vi "CRYUpdate Jump Info Lib.vi"(0 "Steps In":T2[](array[typedef]) {"Repeat State Array"."Start" format="%#_5g"; "Y dB ref" format="%.1f"; "Y data" items=["dB", "Lin"]; "Start" format="%#_5g"}, 1 "sOption":string, 5 "Action":T3(ring), 7 "Step number Selected":i32, 9 "MoveCount":i32, 11 "SourceCount":i32) -> (4 "Steps Out":T2[](array[typedef]) {"Repeat State Array"."Start" format="%#_5g"; "Y dB ref" format="%.1f"; "Y data" items=["dB", "Lin"]; "Start" format="%#_5g"}, 6 "Jump State Out":T1(array[cluster]), 15 "Canceled?":bool)   [LabVIEW 2013]
uses:
  CRYSystem/Typedef Control/CRYStep.ctl
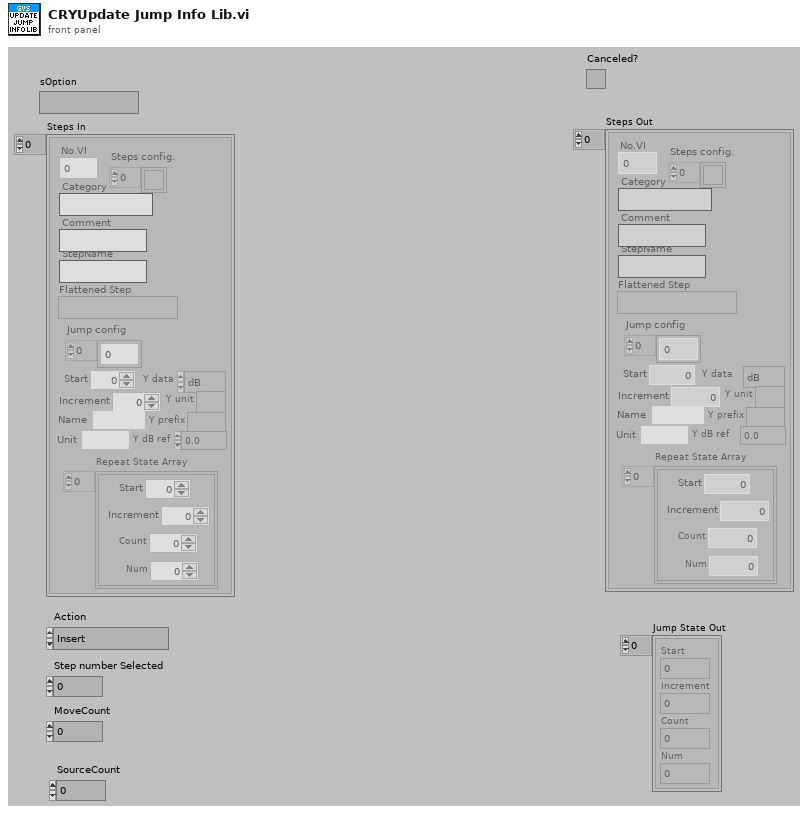
[diagram p1: front panel]
types:
  T1 = cluster{"Start":dbl, "Increment":dbl, "Count":i32, "Num":i32}[]
  T2 = typedef "CRYStep.ctl" = cluster{"No.VI":i32, "Category":string, "StepName":string, "Seq setup flattened":string, "Comment":string, "Steps config.":bool[], "Jump config":i32[], "Start":dbl, "Increment":dbl, "Name":string, "Unit":string, "Y data":u16, "Y prefix":string, "Y dB ref":dbl, "Y unit":string, "Repeat State Array":cluster{"Start":dbl, "Increment":dbl, "Count":i32, "Num":i32}[]}
  T3 = enum16{"Insert", "Remove", "Move up", "Move down"}
  T4 = cluster{"Start":bool, "Increment":bool, "Count":bool, "Num":bool}
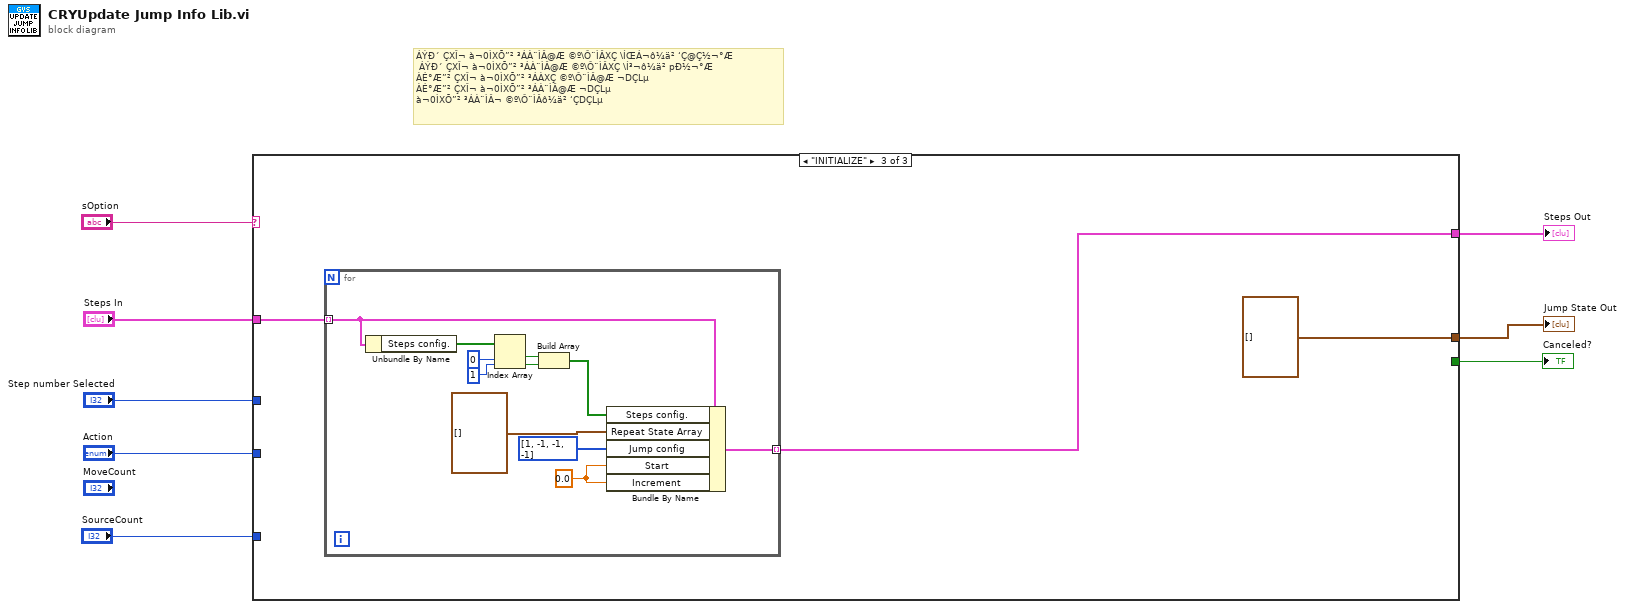
[diagram p0: block diagram]
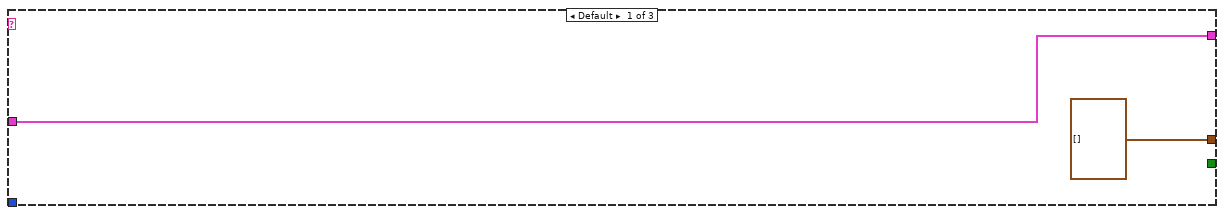
[diagram p2: hidden frame]
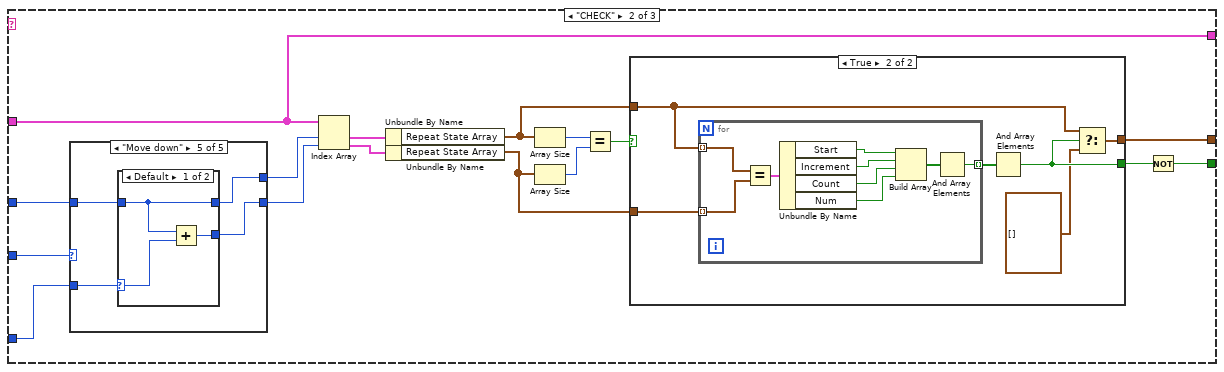
[diagram p3: hidden frame]
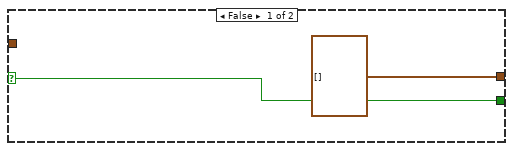
[diagram p4: hidden frame]
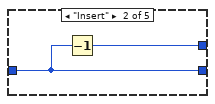
[diagram p6: hidden frame]
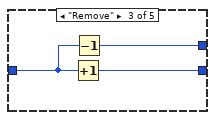
[diagram p7: hidden frame]
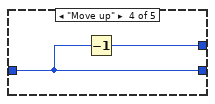
[diagram p8: hidden frame]
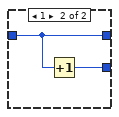
[diagram p9: hidden frame]
diagram:
  # "ÁÝÐ´ ÇXÎ¬ à¬0ÌXÕ”² ³ÁÀ¨ÌÂ@Æ ©º\\Ô¨ÌÂXÇ \\ÍŒÁ¬ô¼ä² ‘Ç@Ç½¬°Æ\n ÁÝÐ´ ÇXÎ¬ à¬0ÌXÕ”² ³ÁÀ¨ÌÂ@Æ ©º\\Ô¨ÌÂXÇ \\Í³¬ô¼ä² pÐ½¬°Æ\nÀÉ°Æ”² ÇXÎ¬ à¬0ÌXÕ”² ³ÁÀXÇ ©º\\Ô¨ÌÂ@Æ ¬DÇLµ\nÀÉ°Æ”² ÇXÎ¬ à¬0ÌXÕ”² ³ÁÀ¨ÌÂ@Æ ¬DÇLµ\nà¬0ÌXÕ”² ³ÁÀ¨ÌÂ¬ ©º\\Ô¨ÌÂô¼ä² ‘ÇDÇLµ"
  n1 = case shown="\"INITIALIZE\"" "sOption" {
    tunnel: "Steps In" -> [w10 w12 w62]
    tunnel: "Action" -> [_ w26 _]
    tunnel: "Step number Selected" -> [_ w25 _]
    tunnel: "SourceCount" -> [_ w15 _]
    tunnel: [_ w13 _] -> w3
    tunnel: [w10 w12 w61] -> w2
    tunnel: [T1 [] ("f") w11 T1 [] ("f")] -> w1
    frame Default {
    }
    frame "CHECK" {
      n2 = case shown="\"Move down\"" w26 {
        tunnel: w25 -> [_ w44 w48 w50 w53]
        tunnel: [_ w45 w47 w49 w52] -> w17
        tunnel: [_ w44 w46 w50 w51] -> w16
        tunnel: w15 -> [_ _ _ _ w54]
        frame Default {
        }
        frame "Insert" {
          n3 = Decrement(x=w44) -> (x-1=w45:i32)
        }
        frame "Remove" {
          n4 = Increment(x=w48) -> (x+1=w46:i32)
          n5 = Decrement(x=w48) -> (x-1=w47:i32)
        }
        frame "Move up" {
          n6 = Decrement(x=w50) -> (x-1=w49:i32)
        }
        frame "Move down" {
          n7 = case shown="Default" w54 {
            selector: w54 -> [w55 _]
            tunnel: [w56 w59] -> w52
            tunnel: w53 -> [w56 w59]
            tunnel: [w57 w58] -> w51
            frame Default {
              n8 = Add(x=w56, y=w55) -> (x+y=w57:i32)
            }
            frame 1 {
              n9 = Increment(x=w59) -> (x+1=w58:i32)
            }
          }
        }
      }
      n10 = Index Array(array=w12, index #1=w17, index #2=w16) -> (element #1=w24:T2, element #2=w23:T2)
      n11 = Unbundle By Name(w24) -> ("Repeat State Array"=w19:T1)
      n12 = Unbundle By Name(w23) -> ("Repeat State Array"=w18:T1)
      n13 = Array Size(array=w19) -> (size(s)=w22:i32)
      n14 = Array Size(array=w18) -> (size(s)=w21:i32)
      n15 = Equal?(x=w22, y=w21) -> (x = y?=w20:bool)
      n16 = case shown="True" w20 {
        selector: w20 -> [w28 _]
        tunnel: w19 -> [_ w31]
        tunnel: w18 -> [_ w34]
        tunnel: [w28 w32] -> w14
        tunnel: [T1 [] ("f") w29] -> w11
        frame False {
        }
        frame True {
          n17 = for {
            tunnel: w31 -> [w43] mode=indexing
            tunnel: w34 -> [w42] mode=indexing
            tunnel: [w35] -> w33 mode=indexing
            n18 = Equal?(x=w43, y=w42) -> (x = y?=w41:T4)
            n19 = Unbundle By Name(w41) -> ("Start"=w40:bool, "Increment"=w39:bool, "Count"=w38:bool, "Num"=w37:bool)
            n20 = Build Array(w40, w39, w38, w37) -> (w36:bool[])
            n21 = And Array Elements(Boolean array=w36) -> (logical AND=w35:bool)
          }
          n22 = And Array Elements(Boolean array=w33) -> (logical AND=w32:bool)
          n23 = Select(t=w31, s=w32, f=T1 []) -> (s? t:f=w29:T1)
        }
      }
      n24 = Not(x=w14) -> (.not. x?=w13:bool)
    }
    frame "INITIALIZE" {
      n25 = for {
        tunnel: w62 -> [w69] mode=indexing
        tunnel: [w70] -> w61 mode=indexing
        w71 = 0.0 ("Start")
        n26 = Unbundle By Name(w69) -> ("Steps config."=w68:bool[])
        n27 = Index Array(array=w68, index #1=0 ("index"), index #2=1 ("index")) -> (element #1=w65:bool, element #2=w64:bool)
        n28 = Build Array(w65, w64) -> (w63:bool[])
        n29 = Bundle By Name(cluster=w69, "Steps config."=w63, "Repeat State Array"=T1 [], "Jump config"=i32[] [1, -1, -1, -1], "Start"=w71, "Increment"=w71) -> (w70:T2)
      }
    }
  }
  "Canceled?" <- w3
  "Steps Out" <- w2
  "Jump State Out" <- w1
